vi "SHOW_CONFIGURATION_DATA.vi"(8 "error in (no error)":errorcluster) -> (0 "error out":errorcluster)   [LabVIEW 2017, in "ZBOX_IS.lvlib"]
uses:
  ZBOX_IS.lvlib
panel:
  out "DLL version":string
  out "Front End":string
  out "Status":string
  out "BinCnt":u16=15
  in  "close":bool
  out "InputCompenValImaginary":sgl[](array[numeric]) format="%.3p"
  out "InputCompenValReal":sgl[](array[numeric])=[1000000000.0, 1000000000.0, 1000000000.0, 1000000000.0, 1000000000.0, 1000000000.0, 1000000000.0, 1000000000.0, 1000000000.0, 1000000000.0, 1000000000.0, 1000000000.0, 1000000000.0, 1000000000.0, 1000000000.0] format="%.3p"
  out "ShuntImpedanceImaginary":sgl[](array[numeric]) format="%.3p"
  out "ShuntImpedanceReal":sgl[](array[numeric])=[1000.0, 1000.0, 1000.0, 1000.0, 1000.0, 1000.0, 1000.0, 1000.0, 1000.0, 1000.0, 1000.0, 1000.0, 1000.0, 1000.0, 1000.0] format="%.3p"
  out "DFTBins":u16[](array[numeric])=[1, 2, 3, 7, 11, 17, 23, 31, 43, 61, 89, 127, 179, 251, 349]
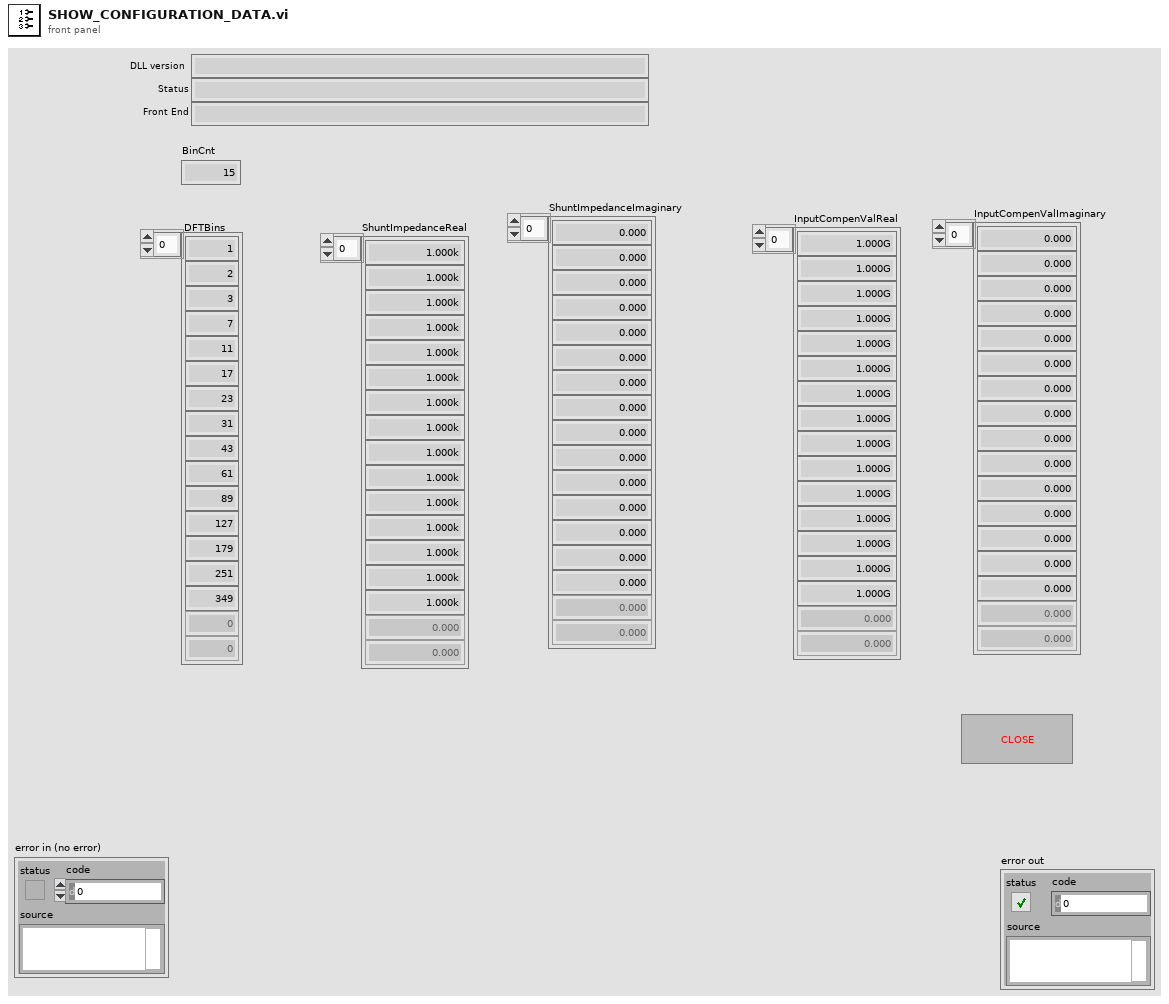
[diagram p1: front panel]
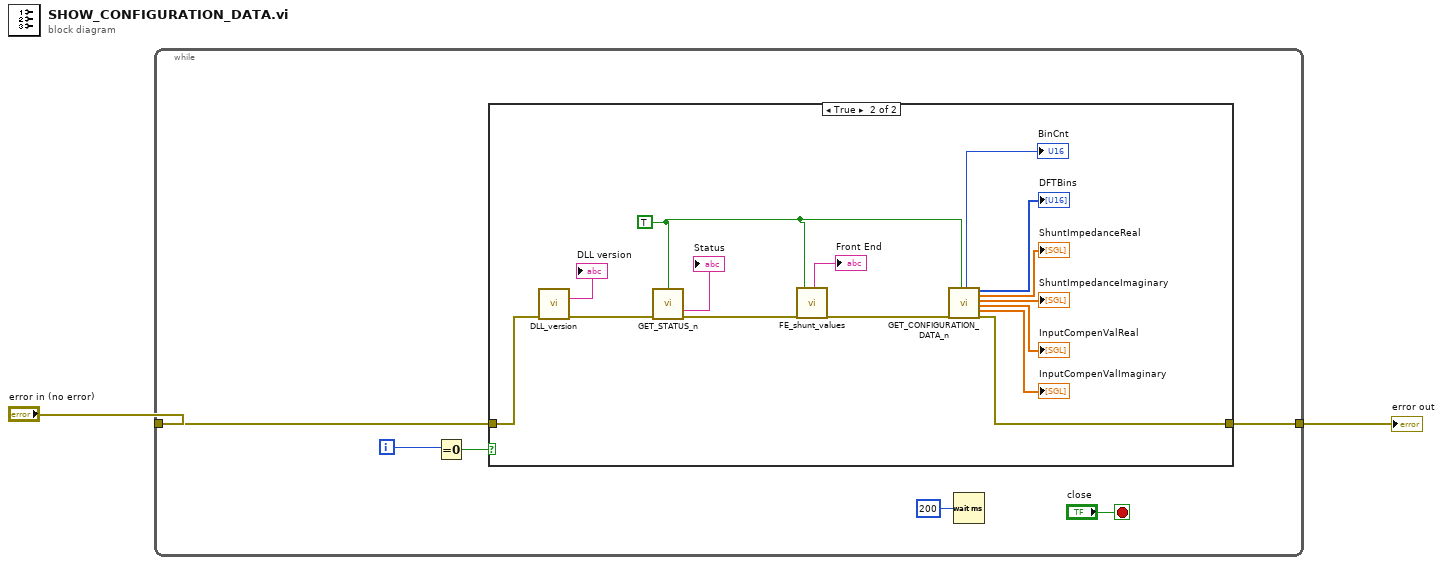
[diagram p0: block diagram]
diagram:
  n1 = while {
    tunnel: "error in (no error)" -> [w4]
    tunnel: [w3] -> w1
    i -> [w5]
    stop <- "close" stop-if-true
    n2 = Equal To 0?(x=w5) -> (x = 0?=w6:bool)
    n3 = case shown="True" w6 {
      tunnel: w4 -> [w9 w12]
      tunnel: [w9 w18] -> w3
      frame False {
      }
      frame True {
        w14 = TRUE ("execute")
        n4 = call "DLL_version.vi"("error in (no error)"=w12) -> ("DLL version"=→"DLL version":string, "error out"=w11:errorcluster)  [unwired: 12 in, 1 out]
        n5 = call "GET_STATUS_n.vi"("execute"=w14, "error in (no error)"=w11) -> ("serial no"=→"Status":string, "error out"=w17:errorcluster)  [unwired: 10 in, 2 out]
        n6 = call "FE_shunt_values.vi"("error in (no error)"=w17, "execute"=w14) -> ("shunt"=→"Front End":string, "error out"=w16:errorcluster)  [unwired: 14 in, 2 out]
        n7 = call "GET_CONFIGURATION_DATA_n.vi"("error in (no error)"=w16, "execute"=w14) -> ("BinCnt"=→"BinCnt":u16, "DFTBins"=→"DFTBins":u16[], "ShuntImpedanceReal"=→"ShuntImpedanceReal":sgl[], "ShuntImpedanceImaginary"=→"ShuntImpedanceImaginary":sgl[], "InputCompenValReal"=→"InputCompenValReal":sgl[], "InputCompenValImaginary"=→"InputCompenValImaginary":sgl[], "error out"=w18:errorcluster)  [unwired: 7 in, 4 out]
      }
    }
    n8 = Wait (ms)(milliseconds to wait=u32 200) -> ()  [unwired: 1 out]
  }
  "error out" <- w1
